vi "real_time.vi"(1 "End time (s)":dbl(slide) scale=0.0..200.0, 2 "FFT interval (s)":dbl(slide)=4.0 scale=0.0..10.0) -> (0 "activity output sensor 1":u16(ring) items=["A", "B", "C", "D", "E", "F"])   [LabVIEW 2009]
panel:
  out "High":bool
  out "Medium":bool
  out "Low":bool
  out "Intensity":dbl(slide) scale=0.0..1.5
  out "max amplitude sensor 3":dbl(slide) scale=0.0..1.5
  out "max amplitude sensor 2":dbl(slide) scale=0.0..1.5
  out "max amplitude sensor 1":dbl(slide) scale=0.0..1.5
  out "D":bool
  out "A":bool
  out "C":bool
  out "B":bool
  out "Activity":u32(ring) items=["A", "B", "C", "D", "E", "F"]
  in  "Controls sensor 3":dbl[](array[slide])=[0.836734693877551, 0.7142857142857142, 0.9081632653061223, 0.8673469387755102] scale=0.0..1.0
  in  "Controls sensor 2":dbl[](array[slide])=[0.8571428571428571, 0.673469387755102, 0.16326530612244897, 0.8265306122448979] scale=0.0..1.0
  in  "Controls sensor 1":dbl[](array[slide])=[0.26530612244897955, 0.3571428571428571, 0.4081632653061224, 0.24489795918367346] scale=0.0..1.0
  out "activity output sensor 3":u16(ring) items=["A", "B", "C", "D", "E", "F"]
  out "activity output sensor 2":u16(ring) items=["A", "B", "C", "D", "E", "F"]
  out "output 3":dbl[](array[slide]) scale=0.0..1.0
  out "output 2":dbl[](array[slide]) scale=0.0..1.0
  in  "stop":bool
  in  "Path":path=path "E:/Sensor/data/Craig walking ADI.csv"
  in  "Sensor Type":u16(ring) items=["Acceleration", "Rotation"]
  in  "Sensor Brand 1":u16(ring) items=["ADXL", "Kinetisense"]
  out "output":dbl[](array[slide]) scale=0.0..1.0
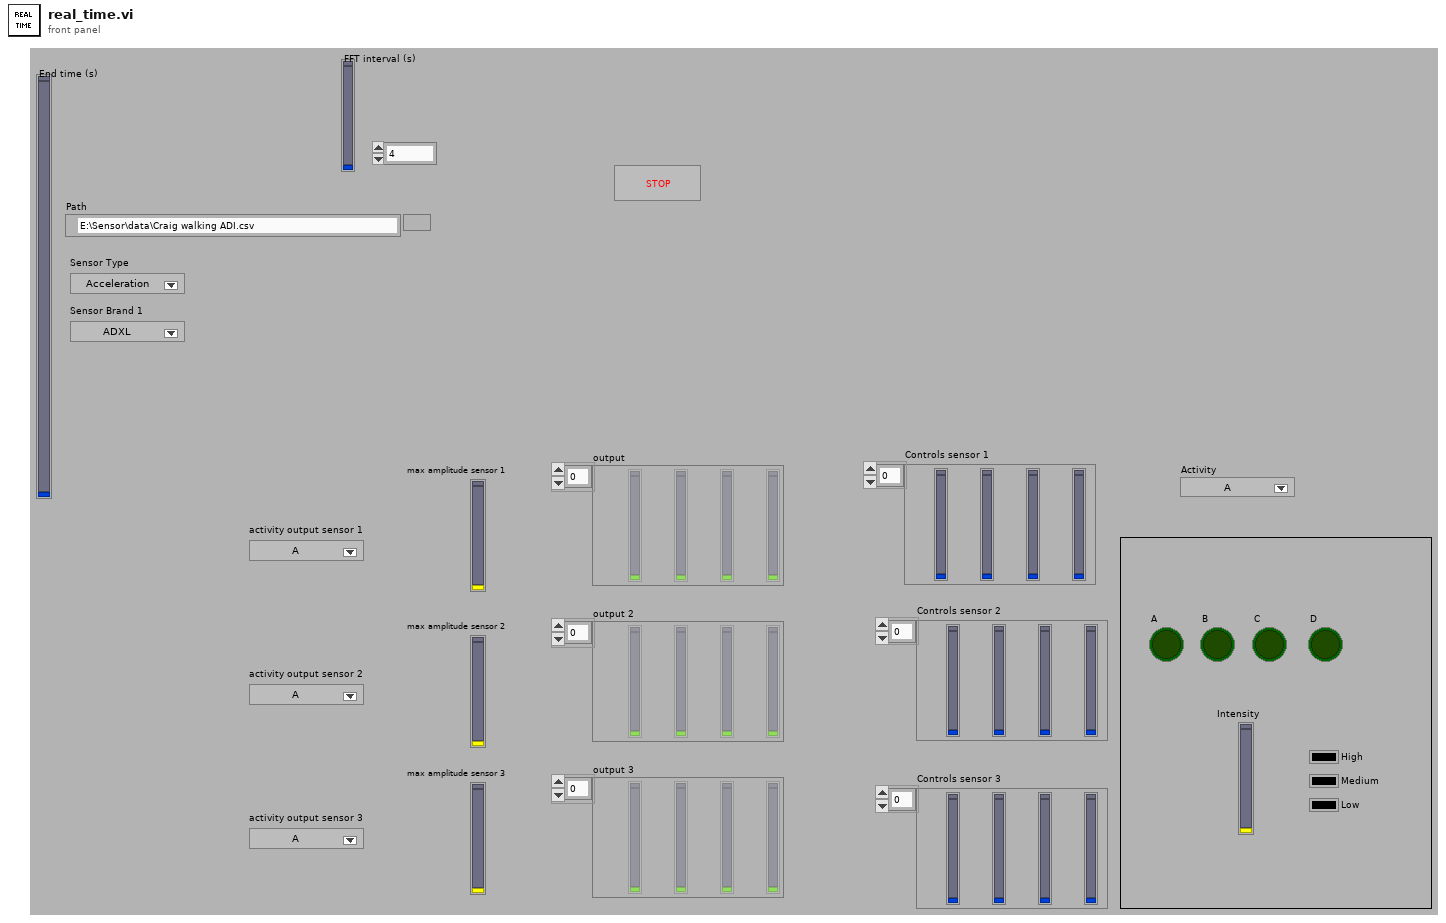
[diagram p1: front panel]
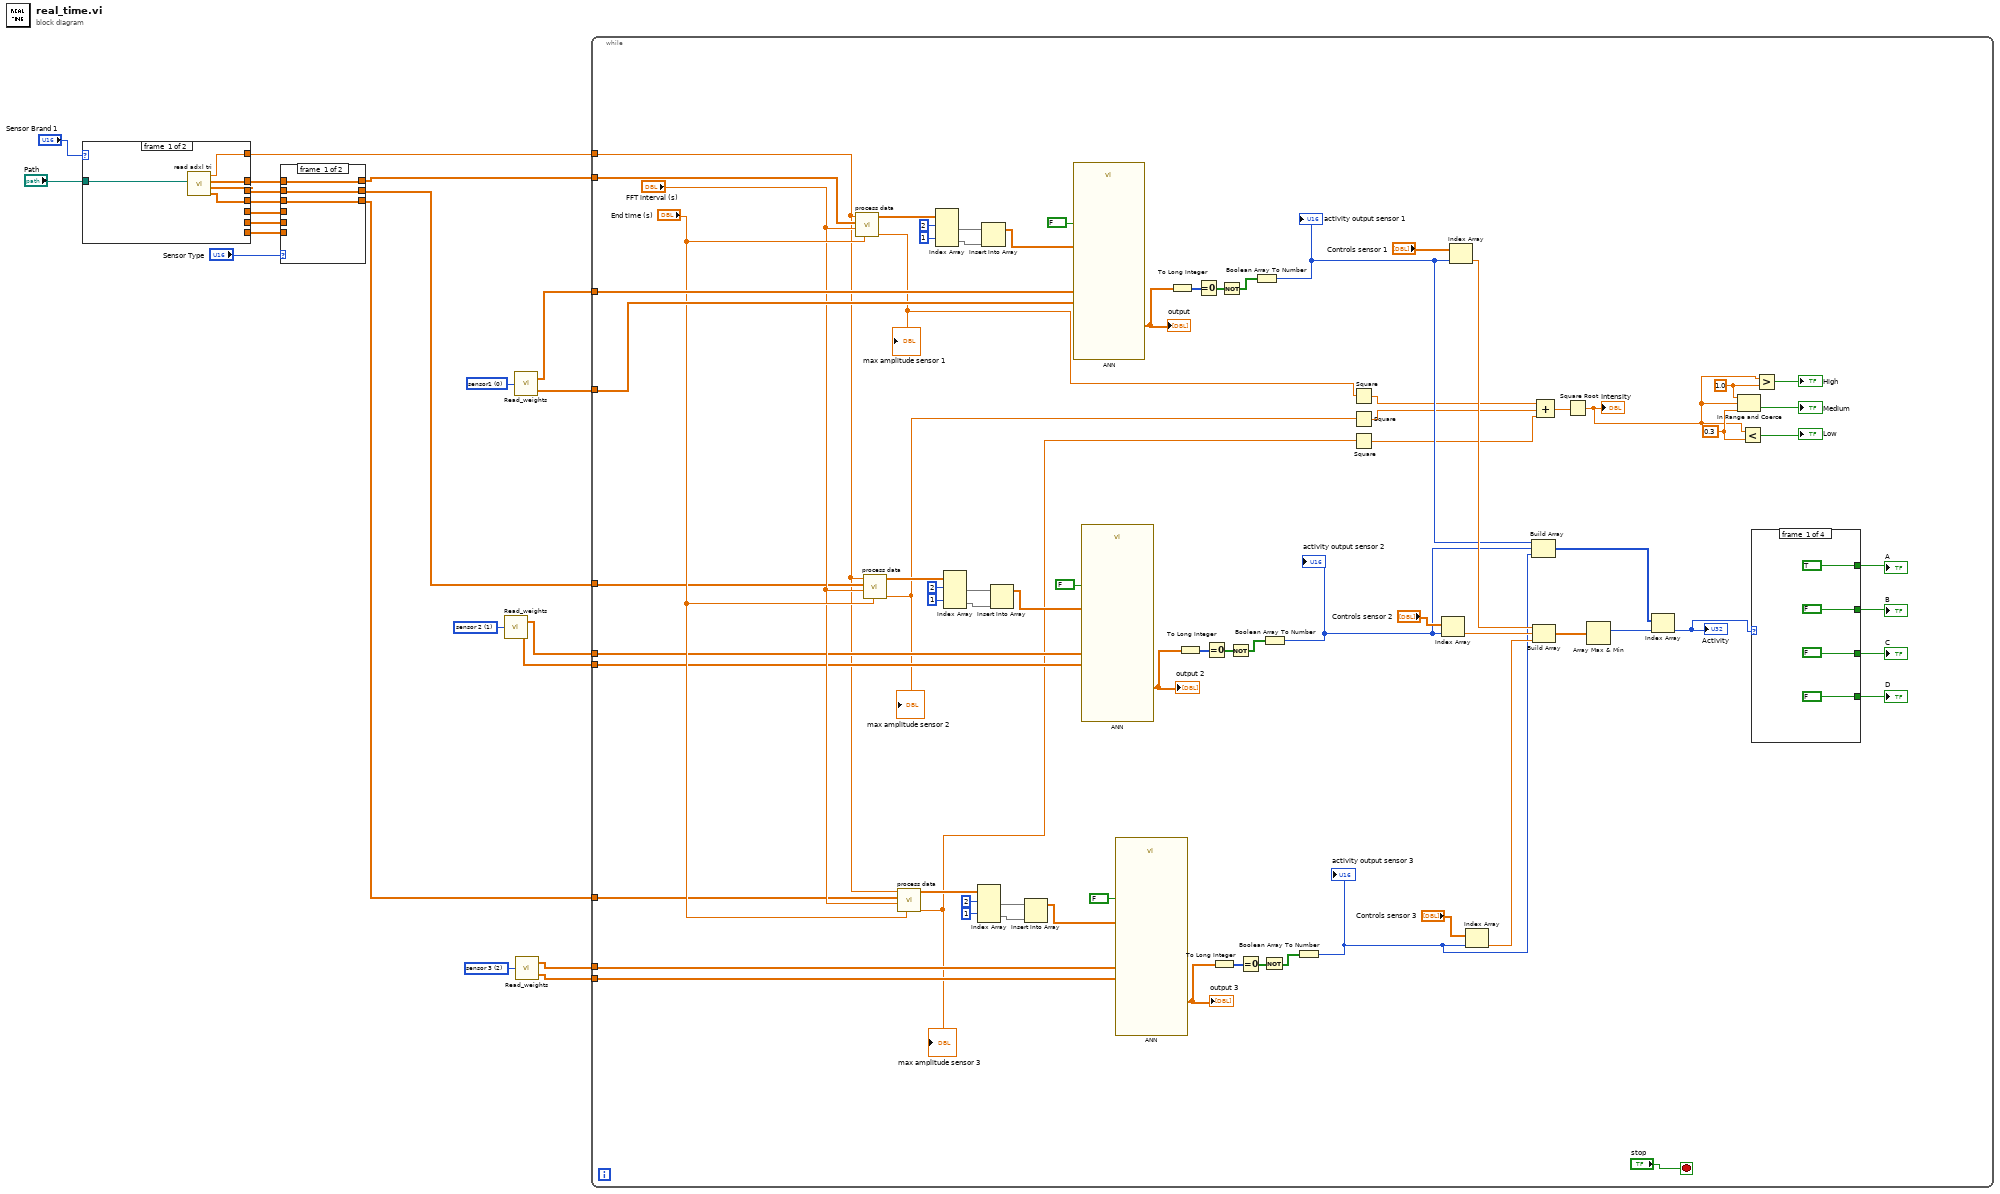
[diagram p0: block diagram]
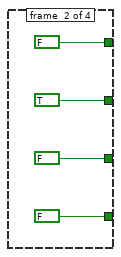
[diagram p2: hidden frame]
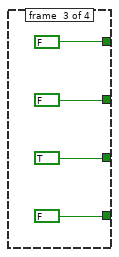
[diagram p3: hidden frame]
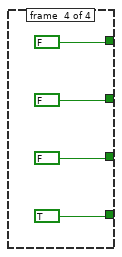
[diagram p4: hidden frame]
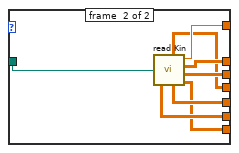
[diagram p6: hidden frame]
diagram:
  w10 = u16 1 items=["sensor1", "sensor 2", "sensor 3"] ("sensor")
  w11 = u16 2 items=["sensor1", "sensor 2", "sensor 3"] ("sensor")
  w12 = u16 0 items=["sensor1", "sensor 2", "sensor 3"] ("sensor")
  n1 = case shown="0, Default" "Sensor Brand 1" {
    tunnel: [w27 w35] -> w13
    tunnel: [w26 w34] -> w21
    tunnel: [w25 w33] -> w22
    tunnel: [w24 w32] -> w20
    tunnel: [_ w31] -> w19
    tunnel: [_ w30] -> w18
    tunnel: [_ w29] -> w17
    tunnel: "Path" -> [w23 w28]
    frame #0 {
      n2 = call "read adxl tri.vi"("file path"=w23) -> ("sensor 3 acceleration"=w24:dbl[][], "sensor 2 acceleration"=w26:dbl[][], "sensor 1 acceleration"=w25:dbl[][], "Frequency (Hz)"=w27:dbl)  [unwired: 4 in]
    }
    frame #1 {
      n3 = call "read Kin.vi"("file path"=w28) -> ("sensor 3 rotation"=w29:dbl[][], "sensor 1 rotation"=w31:dbl[][], "sensor 2 acceleration"=w34:dbl[][], "sensor 1 acceleration"=w33:dbl[][], "sensor 3 acceleration"=w32:dbl[][], "Frequency (Hz)"=w35:dbl, "sensor 2 rotation"=w30:dbl[][])  [unwired: 1 in]
    }
  }
  n4 = case shown="0, Default" "Sensor Type" {
    tunnel: w22 -> [w38 _]
    tunnel: w21 -> [w37 _]
    tunnel: w20 -> [w36 _]
    tunnel: w19 -> [_ w41]
    tunnel: w18 -> [_ w40]
    tunnel: w17 -> [_ w39]
    tunnel: [w38 w41] -> w7
    tunnel: [w37 w40] -> w6
    tunnel: [w36 w39] -> w3
    frame #0 {
    }
    frame #1 {
    }
  }
  n5 = call "Read_weights.vi"("sensor"=w10) -> ("weights 1"=w5:dbl[][], "weights 2"=w4:dbl[][])
  n6 = call "Read_weights.vi"("sensor"=w12) -> ("weights 1"=w9:dbl[][], "weights 2"=w8:dbl[][])
  n7 = call "Read_weights.vi"("sensor"=w11) -> ("weights 1"=w2:dbl[][], "weights 2"=w1:dbl[][])
  n8 = while {
    tunnel: w13 -> [w74]
    tunnel: w9 -> [w105]
    tunnel: w8 -> [w104]
    tunnel: w7 -> [w79]
    tunnel: w6 -> [w78]
    tunnel: w5 -> [w77]
    tunnel: w4 -> [w76]
    tunnel: w3 -> [w75]
    tunnel: w2 -> [w73]
    tunnel: w1 -> [w72]
    stop <- "stop" stop-if-true
    w43 = 1.0 ("upper limit")
    w46 = 0.3 ("y")
    n9 = call "process data.vi"("End time (s)"="End time (s)", "FFT interval (s)"="FFT interval (s)", "sensor input"=w79, "Frequency (Hz)"=w74) -> ("max amplitude"=w54:dbl, "peaks"=w107:dbl[][])  [unwired: 1 in, 5 out]
    "max amplitude sensor 1" <- w54
    n10 = call "process data.vi"("End time (s)"="End time (s)", "FFT interval (s)"="FFT interval (s)", "sensor input"=w78, "Frequency (Hz)"=w74) -> ("max amplitude"=w53:dbl, "peaks"=w93:dbl[][])  [unwired: 1 in, 5 out]
    "max amplitude sensor 2" <- w53
    n11 = call "process data.vi"("End time (s)"="End time (s)", "FFT interval (s)"="FFT interval (s)", "sensor input"=w75, "Frequency (Hz)"=w74) -> ("max amplitude"=w52:dbl, "peaks"=w82:dbl[][])  [unwired: 1 in, 5 out]
    "max amplitude sensor 3" <- w52
    n12 = Index Array(array=w107, index (row) #1=2 ("index (row)"), index (row) #2=1 ("index (row)")) -> (element #1=w114:dbl[], element #2=w113:dbl[])  [unwired: 2 in]
    n13 = Index Array(array=w93, index (row) #1=2 ("index (row)"), index (row) #2=1 ("index (row)")) -> (element #1=w100:dbl[], element #2=w99:dbl[])  [unwired: 2 in]
    n14 = Index Array(array=w82, index (row) #1=2 ("index (row)"), index (row) #2=1 ("index (row)")) -> (element #1=w89:dbl[], element #2=w88:dbl[])  [unwired: 2 in]
    n15 = Insert Into Array(array=w114, new element=w113) -> (w112:dbl[])  [unwired: 1 in]
    n16 = Insert Into Array(array=w100, new element=w99) -> (w98:dbl[])  [unwired: 1 in]
    n17 = Insert Into Array(array=w89, new element=w88) -> (w87:dbl[])  [unwired: 1 in]
    n18 = call "ANN.vi"("Input"=w112, "Weight_2"=w104, "Weight_1"=w105, "Back Propagation"=FALSE) -> ("output"=w111:dbl[])  [unwired: 8 in, 3 out]
    "output" <- w111
    n19 = call "ANN.vi"("Input"=w98, "Weight_2"=w76, "Weight_1"=w77, "Back Propagation"=FALSE) -> ("output"=w97:dbl[])  [unwired: 8 in, 3 out]
    "output 2" <- w97
    n20 = call "ANN.vi"("Input"=w87, "Weight_2"=w72, "Weight_1"=w73, "Back Propagation"=FALSE) -> ("output"=w86:dbl[])  [unwired: 8 in, 3 out]
    "output 3" <- w86
    n21 = To Long Integer(number=w111) -> (32bit integer=w110:i32[])
    n22 = To Long Integer(number=w97) -> (32bit integer=w96:i32[])
    n23 = Equal To 0?(x=w110) -> (x = 0?=w109:bool[])
    n24 = Equal To 0?(x=w96) -> (x = 0?=w95:bool[])
    n25 = To Long Integer(number=w86) -> (32bit integer=w85:i32[])
    n26 = Not(x=w109) -> (.not. x?=w108:bool[])
    n27 = Not(x=w95) -> (.not. x?=w94:bool[])
    n28 = Equal To 0?(x=w85) -> (x = 0?=w84:bool[])
    n29 = Boolean Array To Number(Boolean array=w108) -> (number=w64:u32)
    "activity output sensor 1" <- w64
    n30 = Not(x=w84) -> (.not. x?=w83:bool[])
    n31 = Boolean Array To Number(Boolean array=w94) -> (number=w63:u32)
    "activity output sensor 2" <- w63
    n32 = Boolean Array To Number(Boolean array=w83) -> (number=w62:u32)
    "activity output sensor 3" <- w62
    n33 = Square(x=w54) -> (x^2=w51:dbl)
    n34 = Square(x=w53) -> (x^2=w50:dbl)
    n35 = Square(x=w52) -> (x^2=w49:dbl)
    n36 = Index Array(array="Controls sensor 2", index=w63) -> (element=w67:dbl)
    n37 = Index Array(array="Controls sensor 1", index=w64) -> (element=w68:dbl)
    n38 = Index Array(array="Controls sensor 3", index=w62) -> (element=w66:dbl)
    n39 = Build Array(w64, w63, w62) -> (w61:u32[])
    n40 = Build Array(w68, w67, w66) -> (w65:dbl[])
    n41 = Compound Arithmetic op=ADD(w51, w50, w49) -> (w48:dbl)
    n42 = Square Root(x=w48) -> (sqrt(x)=w42:dbl)
    "Intensity" <- w42
    n43 = Array Max & Min(array=w65) -> (max index (indices)=w60:i32)  [unwired: 3 out]
    n44 = Index Array(array=w61, index=w60) -> (element=w59:u32)
    "Activity" <- w59
    n45 = In Range and Coerce(upper limit=w43, x=w42, lower limit=w46) -> (In Range?=→"Medium":bool)  [unwired: 1 out]
    n46 = Less?(x=w42, y=w46) -> (x < y?=→"Low":bool)
    n47 = case shown="0, Default" w59 {
      tunnel: [TRUE FALSE FALSE FALSE] -> w58
      tunnel: [FALSE TRUE FALSE FALSE] -> w57
      tunnel: [FALSE FALSE TRUE FALSE] -> w56
      tunnel: [FALSE FALSE FALSE TRUE] -> w55
      frame #0 {
      }
      frame #1 {
      }
      frame #2 {
      }
      frame #3 {
      }
    }
    "B" <- w57
    "C" <- w56
    "A" <- w58
    "D" <- w55
    n48 = Greater?(x=w42, y=w43) -> (0:→"High":bool)
  }
